vi "SetMultipleTilesByCode.vi"(8 "error in (no error)":errorcluster, 9 "Position":T1, 10 "TileCodes":u32[][](array[numeric]), 11 "Game in":refnum<class "Game.lvclass">) -> (0 "error out":errorcluster, 3 "Game out":refnum<class "Game.lvclass">)   [LabVIEW 2019, in "RT_Game.lvlib" / "Game.lvclass"]
uses:
  Game.lvclass
  Coordinate.ctl
  Game.lvclass/Game.ctl
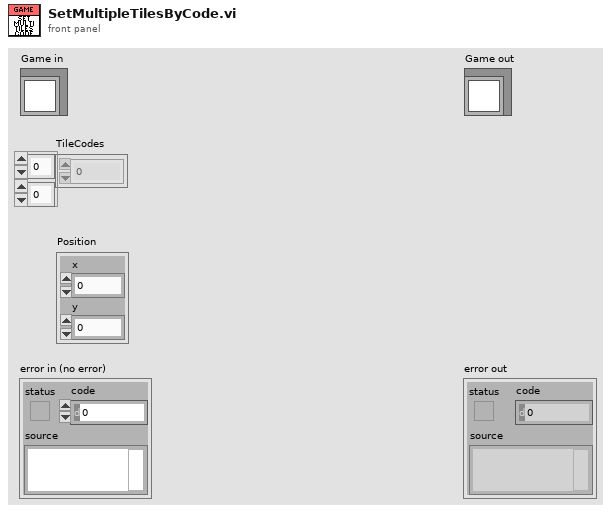
[diagram p1: front panel]
types:
  T1 = typedef "RT_Game.lvlib/Game.lvclass/Coordinate.ctl" = cluster{"x":dbl, "y":dbl}
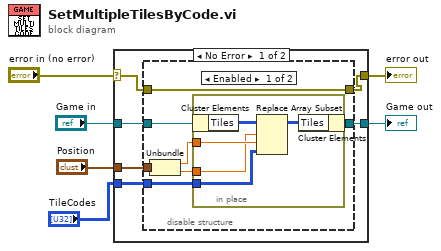
[diagram p0: block diagram]
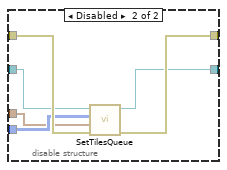
[diagram p2: hidden frame]
diagram:
  n1 = case shown="No Error" "error in (no error)" {
    selector: "error in (no error)" -> [w8 w32]
    tunnel: [w7 w32] -> w1
    tunnel: [w9 w31] -> w5
    tunnel: "Game in" -> [w10 w31]
    tunnel: "Position" -> [w12 _]
    tunnel: "TileCodes" -> [w11 _]
    frame No Error {
      n2 = disable-structure shown="Enabled" {
        disable-tunnel: w12 -> [w19 w25]
        disable-tunnel: w11 -> [w18 w26]
        disable-tunnel: w10 -> [w17 w28]
        disable-tunnel: [w16 w27] -> w9
        disable-tunnel: w8 -> [w13 w30]
        disable-tunnel: [w13 w29] -> w7
        frame Enabled {
          n3 = Unbundle(w19) -> ("x"=w15:dbl, "y"=w14:dbl)
          n4 = in-place {
            in-place-border: w15 -> [w24]
            in-place-border: w14 -> [w23]
            in-place-border: w18 -> [w22]
            n5 = in-place-cluster #1(w17) -> ("Tiles"=w20:u32[][])
            n6 = Replace Array Subset(array=w20, new element=w22, index (row)=w23, index (col)=w24) -> (w21:u32[][])
            n7 = in-place-cluster #1("Tiles"=w21) -> (w16:refnum<class "Game.lvclass">)
          }
        }
        frame Disabled {
          n8 = call "SetTilesQueue.vi"("error in (no error)"=w30, "Position"=w25, "TileCodes"=w26, "Game in"=w28) -> ("error out"=w29:errorcluster, "Game out"=w27:refnum<class "Game.lvclass">)  [unwired: 6 in]
        }
      }
    }
    frame Error {
    }
  }
  "error out" <- w1
  "Game out" <- w5
